vi "Detect Hit Step Counter.vi"(9 "Base Step":i32, 10 "millisecond timer value in":u32, 11 "Step":i32) -> (2 "t out":dbl, 3 "millisecond timer value out":u32)   [LabVIEW 2016]
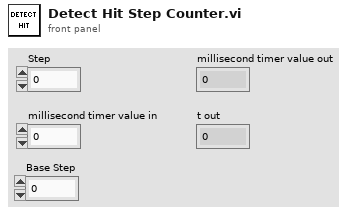
[diagram p1: front panel]
types:
  T1 = cluster{"LinearAcceleration X":dbl, "LinearAcceleration Y":dbl, "LinearAcceleration Z":dbl}
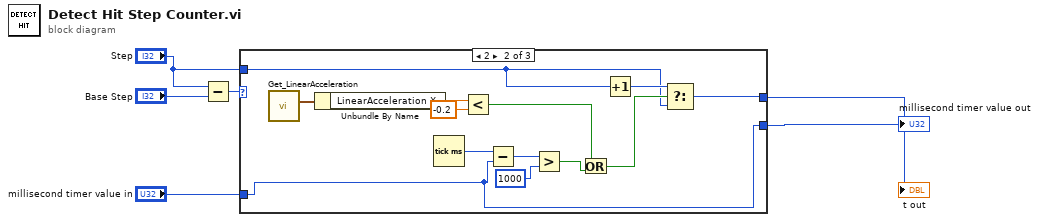
[diagram p0: block diagram]
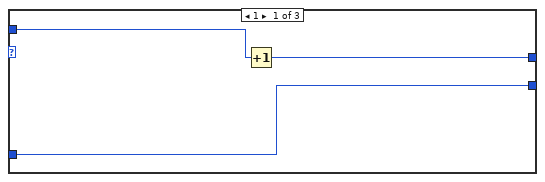
[diagram p2: hidden frame]
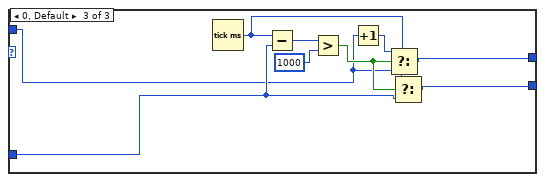
[diagram p3: hidden frame]
diagram:
  n1 = Subtract(x="Step", y="Base Step") -> (x-y=w3:i32)
  n2 = case shown="2" w3 {
    tunnel: [w8 w14 w24] -> w5
    tunnel: "millisecond timer value in" -> [w8 w14 w25]
    tunnel: [w9 w19 w28] -> w4
    tunnel: "Step" -> [w7 w10 w23]
    frame 1 {
      n3 = Increment(x=w7) -> (x+1=w9:i32)
    }
    frame 2 {
      n4 = call <vilib>:"Get_LinearAcceleration.vi"() -> ("Linear Acceleration"=w22:T1)  [unwired: 11 in]
      n5 = Unbundle By Name(w22) -> ("LinearAcceleration X"=w21:dbl)
      n6 = Tick Count (ms)() -> (millisecond timer value=w17:u32)
      n7 = Less?(x=w21, y=-0.2) -> (x < y?=w12:bool)
      n8 = Subtract(x=w17, y=w14) -> (x-y=w16:u32)
      n9 = Greater?(x=w16, y=u32 1000) -> (0:w13:bool)
      n10 = Or(x=w12, y=w13) -> (x .or. y?=w11:bool)
      n11 = Increment(x=w10) -> (x+1=w18:i32)
      n12 = Select(t=w18, s=w11, f=w10) -> (s? t:f=w19:i32)
    }
    frame 0, Default {
      n13 = Tick Count (ms)() -> (millisecond timer value=w26:u32)
      n14 = Subtract(x=w26, y=w25) -> (x-y=w31:u32)
      n15 = Greater?(x=w31, y=u32 1000) -> (0:w27:bool)
      n16 = Increment(x=w23) -> (x+1=w29:i32)
      n17 = Select(t=w29, s=w27, f=w23) -> (s? t:f=w28:i32)
      n18 = Select(t=w26, s=w27, f=w25) -> (s? t:f=w24:u32)
    }
  }
  "millisecond timer value out" <- w5
  "t out" <- w4
